vi "SLM_Azimuthal Generation.vi"(1 "p":i16 min=0 step=1, 2 "l":i16, 3 "beam parameters":T1={"amplitude matrix"=[], "number of columns in amplitude matrix"=128, "number of rows in amplitude matrix"=128, "represented width (in m)"=0.001, "represented height (in m)"=0.001, "wavelength (in m)"=6.33e-07} {"wavelength (in m)" format="%.2p"; "represented height (in m)" format="%.2p"; "represented width (in m)" format="%.2p"; "amplitude matrix" format="%.2f"}) -> (0 "Laguerre-Gaussian beam":T1 {"wavelength (in m)" format="%.2f"; "represented height (in m)" format="%.2f"; "represented width (in m)" format="%.2f"; "amplitude matrix" format="%.2f"})   [LabVIEW 2024]
panel:
  in  "y centre":dbl
  in  "x centre":dbl
  out "max value":dbl
  out "min value":dbl
  in  "beam waist w0 (in m; default 1E-4 = 0.1mm)":dbl=0.0001 format="%.2p"
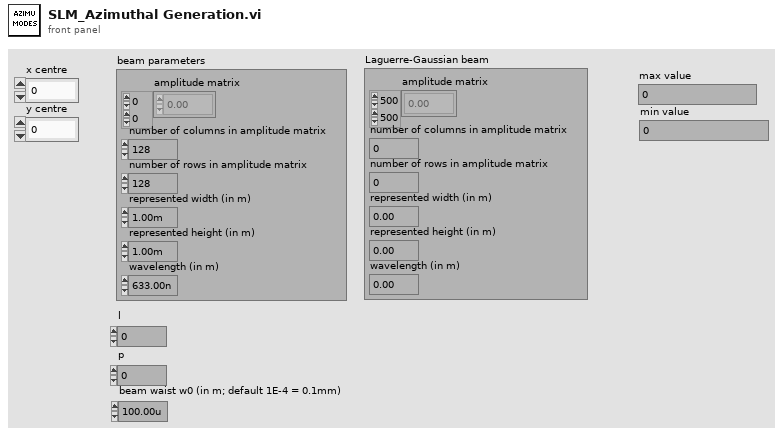
[diagram p1: front panel]
types:
  T1 = cluster{"amplitude matrix":csg[][], "number of columns in amplitude matrix":i32, "number of rows in amplitude matrix":i32, "represented width (in m)":dbl, "represented height (in m)":dbl, "wavelength (in m)":dbl}
  T2 = cluster{"x values":dbl[], "laguerre polynomial values":dbl[]}
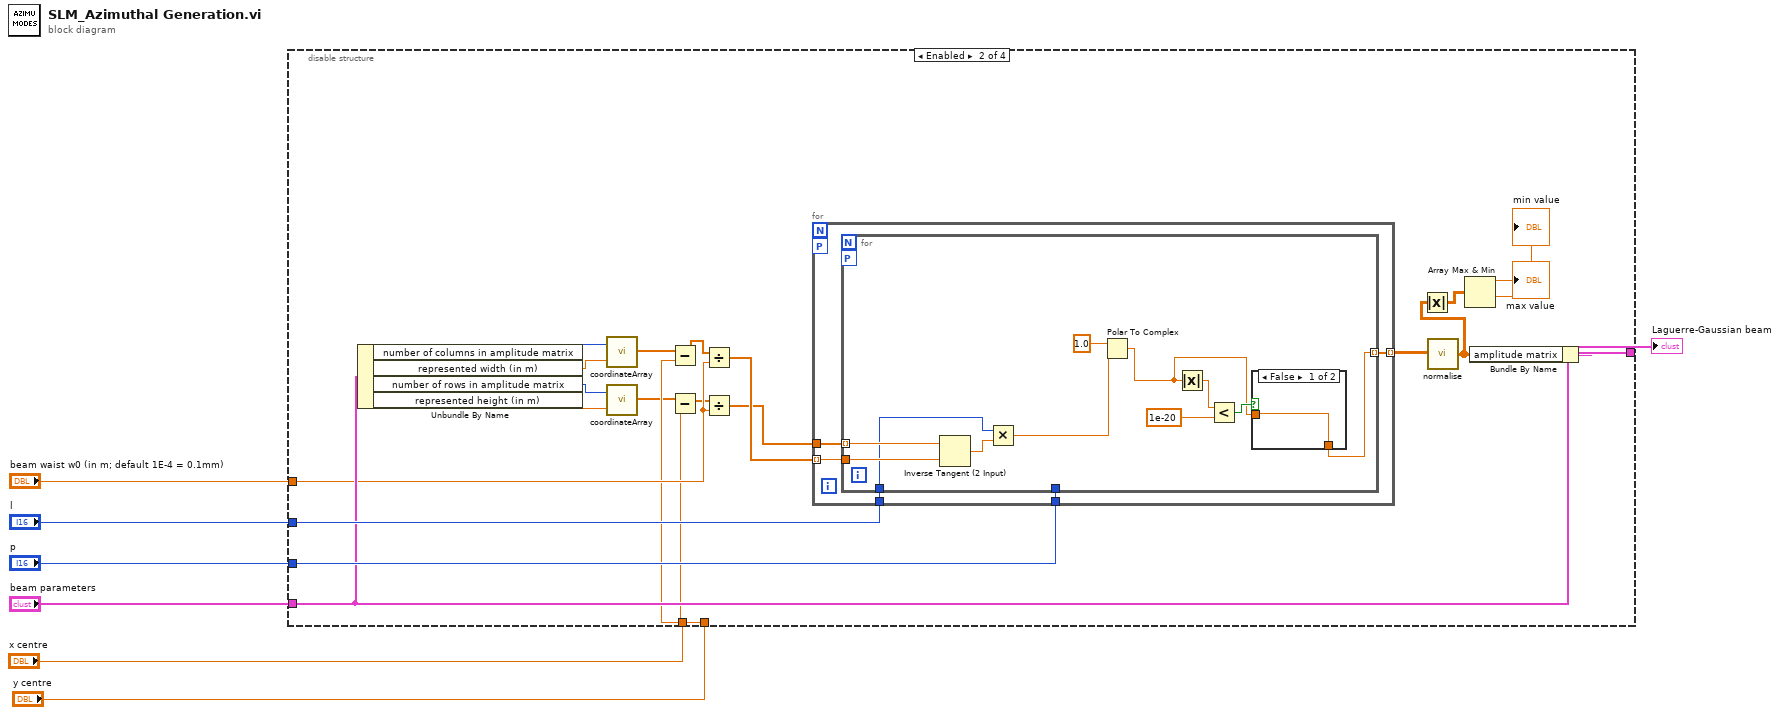
[diagram p0: block diagram]
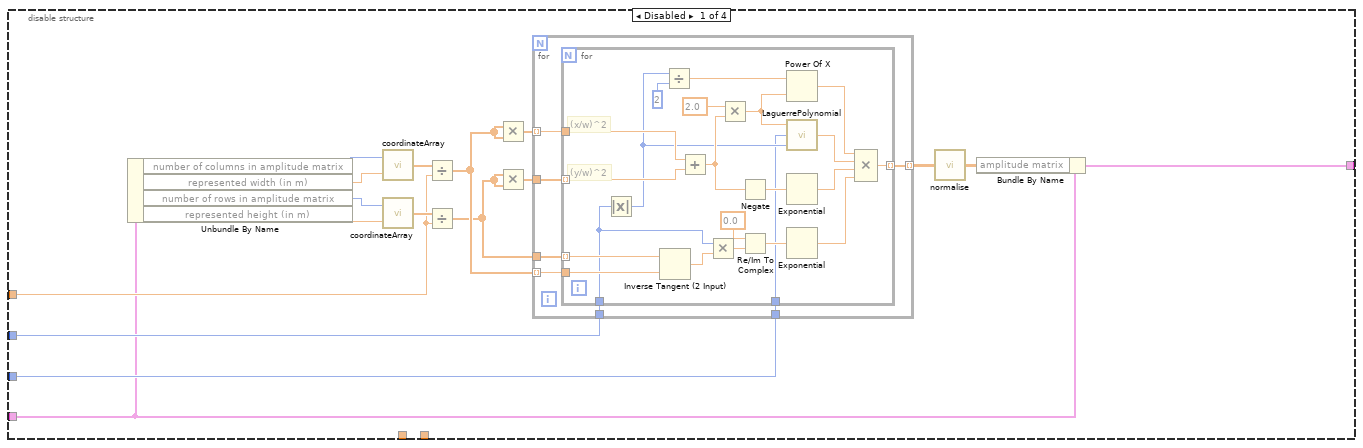
[diagram p2: hidden frame]
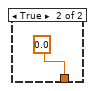
[diagram p3: hidden frame]
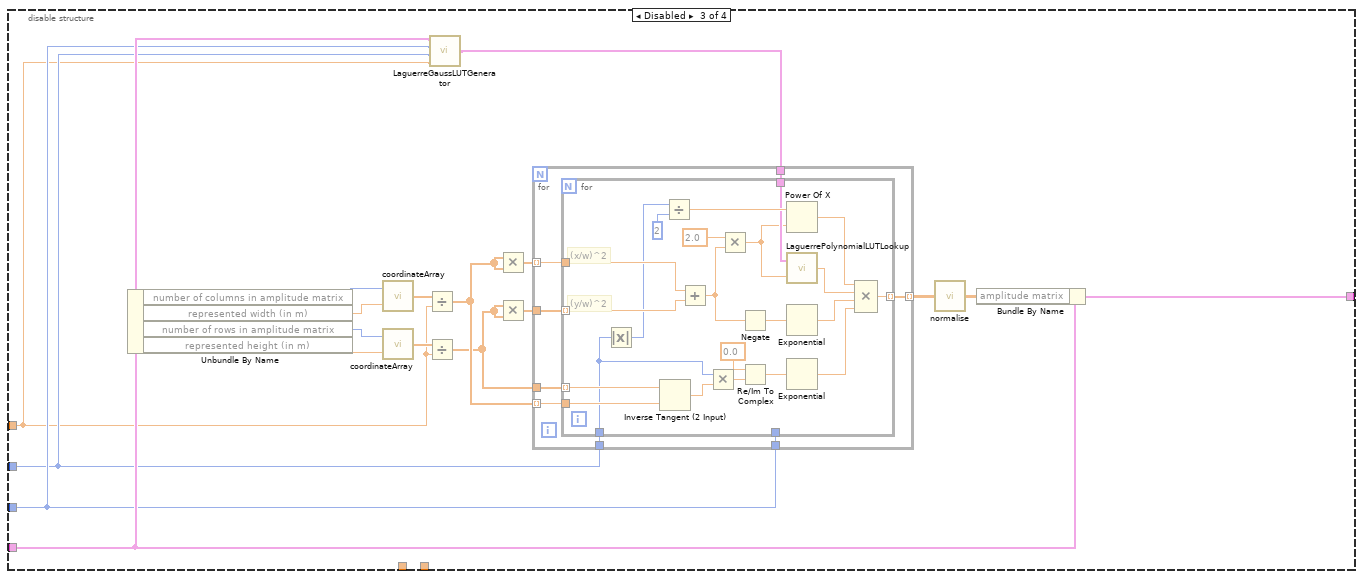
[diagram p4: hidden frame]
diagram:
  n1 = disable-structure shown="Enabled" {
    disable-tunnel: [w24 w75 w111 _] -> w7
    disable-tunnel: "p" -> [w11 w70 w96 _]
    disable-tunnel: "l" -> [w10 w69 w95 _]
    disable-tunnel: "beam waist w0 (in m; default 1E-4 = 0.1mm)" -> [w9 w67 w94 _]
    disable-tunnel: "beam parameters" -> [w8 w68 w97 _]
    disable-tunnel: "x centre" -> [_ w65 _ _]
    disable-tunnel: "y centre" -> [_ w66 _ _]
    frame Disabled {
      n2 = Unbundle By Name(w8) -> ("number of columns in amplitude matrix"=w23:i32, "represented width (in m)"=w13:dbl, "number of rows in amplitude matrix"=w22:i32, "represented height (in m)"=w12:dbl)
      n3 = call "coordinateArray.vi"("width of represented x (or y) range (in m; default 1E-3=1mm)"=w13, "array size (default 64)"=w23) -> ("x array"=w21:sgl[])
      n4 = call "coordinateArray.vi"("width of represented x (or y) range (in m; default 1E-3=1mm)"=w12, "array size (default 64)"=w22) -> ("x array"=w20:sgl[])
      n5 = Divide(x=w21, y=w9) -> (x/y=w17:dbl[])
      n6 = Divide(x=w20, y=w9) -> (x/y=w16:dbl[])
      n7 = Multiply(x=w17, y=w17) -> (x*y=w19:dbl[])
      n8 = Multiply(x=w16, y=w16) -> (x*y=w18:dbl[])
      n9 = for {
        tunnel: [w31] -> w15 mode=indexing
        tunnel: w19 -> [w30] mode=indexing
        tunnel: w18 -> [w29]
        tunnel: w17 -> [w28] mode=indexing
        tunnel: w16 -> [w27]
        tunnel: w10 -> [w26]
        tunnel: w11 -> [w25]
        n10 = for {
          tunnel: [w52] -> w31 mode=indexing
          tunnel: w30 -> [w51]
          tunnel: w29 -> [w50] mode=indexing
          tunnel: w28 -> [w40]
          tunnel: w27 -> [w39] mode=indexing
          tunnel: w26 -> [w36]
          tunnel: w25 -> [w32]
          # "(y/w)^2"
          # "(x/w)^2"
          n11 = Absolute Value(x=w36) -> (abs(x)=w33:i16)
          n12 = Inverse Tangent (2 Input)(1:w40, 2:w39) -> (0:w43:dbl)
          n13 = Divide(x=w33, y=i16 2) -> (x/y=w37:dbl)
          n14 = Add(x=w51, y=w50) -> (x+y=w47:dbl)
          n15 = Multiply(x=w36, y=w43) -> (x*y=w44:dbl)
          n16 = Multiply(x=2.0, y=w47) -> (x*y=w34:dbl)
          n17 = Negate(x=w47) -> (-x=w53:dbl)
          n18 = Re/Im To Complex(1:w44, 2:0.0 ("x")) -> (0:w45:cdb)
          n19 = Power Of X(1:w34, 2:w37) -> (0:w48:dbl)
          n20 = call "LaguerrePolynomial.vi"("a"=w33, "n"=w32, "x"=w34) -> ("associated Laguerre polynomial (n,a,x)"=w35:dbl)
          n21 = Exponential(1:w53) -> (0:w46:dbl)
          n22 = Exponential(1:w45) -> (0:w41:cdb)
          n23 = Compound Arithmetic op=MULTIPLY(w48, w35, w46, w41) -> (w52:cdb)
        }
      }
      n24 = call "normalise.vi"("amplitude matrix"=w15) -> ("normalised amplitude matrix"=w14:cdb[][])
      n25 = Bundle By Name(cluster=w8, "amplitude matrix"=w14) -> (w24:T1)
    }
    frame Enabled {
      n26 = Unbundle By Name(w68) -> ("number of columns in amplitude matrix"=w74:i32, "represented width (in m)"=w72:dbl, "number of rows in amplitude matrix"=w73:i32, "represented height (in m)"=w71:dbl)
      n27 = call "coordinateArray.vi"("width of represented x (or y) range (in m; default 1E-3=1mm)"=w72, "array size (default 64)"=w74) -> ("x array"=w64:sgl[])
      n28 = call "coordinateArray.vi"("width of represented x (or y) range (in m; default 1E-3=1mm)"=w71, "array size (default 64)"=w73) -> ("x array"=w61:sgl[])
      n29 = Subtract(x=w64, y=w65) -> (x-y=w60:dbl[])
      n30 = Subtract(x=w61, y=w66) -> (x-y=w59:dbl[])
      n31 = Divide(x=w60, y=w67) -> (x/y=w63:dbl[])
      n32 = Divide(x=w59, y=w67) -> (x/y=w62:dbl[])
      n33 = for {
        tunnel: [w80] -> w54 mode=indexing
        tunnel: w63 -> [w79] mode=indexing
        tunnel: w62 -> [w78]
        tunnel: w69 -> [w77]
        tunnel: w70 -> [w76]
        workers-P: _ -> [_]
        n34 = for {
          tunnel: [w83] -> w80 mode=indexing
          tunnel: w79 -> [w90]
          tunnel: w78 -> [w89] mode=indexing
          tunnel: w77 -> [w88]
          tunnel: w76 -> [_]
          workers-P: _ -> [_]
          n35 = Inverse Tangent (2 Input)(1:w90, 2:w89) -> (0:w91:dbl)
          n36 = Multiply(x=w88, y=w91) -> (x*y=w87:dbl)
          n37 = Polar To Complex(1:w87, 2:1.0 ("r")) -> (0:w81:cdb)
          n38 = Absolute Value(x=w81) -> (abs(x)=w86:dbl)
          n39 = Less?(x=w86, y=1e-20) -> (x < y?=w84:bool)
          n40 = case shown="False" w84 {
            tunnel: w81 -> [w92 _]
            tunnel: [w92 0.0 ("y")] -> w83
            frame False {
            }
            frame True {
            }
          }
        }
      }
      n41 = call "normalise.vi"("amplitude matrix"=w54) -> ("normalised amplitude matrix"=w55:cdb[][])
      n42 = Absolute Value(x=w55) -> (abs(x)=w58:dbl[][])
      n43 = Array Max & Min(array=w58) -> (max value=→"max value":dbl, min value=→"min value":dbl)  [unwired: 2 out]
      n44 = Bundle By Name(cluster=w68, "amplitude matrix"=w55) -> (w75:T1)
    }
    frame Disabled {
      n45 = Unbundle By Name(w97) -> ("number of columns in amplitude matrix"=w110:i32, "represented width (in m)"=w100:dbl, "number of rows in amplitude matrix"=w109:i32, "represented height (in m)"=w99:dbl)
      n46 = call "coordinateArray.vi"("width of represented x (or y) range (in m; default 1E-3=1mm)"=w100, "array size (default 64)"=w110) -> ("x array"=w108:sgl[])
      n47 = call "coordinateArray.vi"("width of represented x (or y) range (in m; default 1E-3=1mm)"=w99, "array size (default 64)"=w109) -> ("x array"=w107:sgl[])
      n48 = Divide(x=w108, y=w94) -> (x/y=w104:dbl[])
      n49 = Divide(x=w107, y=w94) -> (x/y=w103:dbl[])
      n50 = call "LaguerreGaussLUTGenerator.vi"("beam waist w0 (in m; default 1E-4 = 0.1mm)"=w94, "l"=w95, "p"=w96, "beam parameters"=w97) -> ("Look-up Table"=w98:T2)
      n51 = Multiply(x=w104, y=w104) -> (x*y=w106:dbl[])
      n52 = Multiply(x=w103, y=w103) -> (x*y=w105:dbl[])
      n53 = for {
        tunnel: [w119] -> w102 mode=indexing
        tunnel: w106 -> [w118] mode=indexing
        tunnel: w105 -> [w117]
        tunnel: w104 -> [w116] mode=indexing
        tunnel: w103 -> [w115]
        tunnel: w95 -> [w114]
        tunnel: w96 -> [w113]
        tunnel: w98 -> [w112]
        n54 = for {
          tunnel: [w140] -> w119 mode=indexing
          tunnel: w118 -> [w139]
          tunnel: w117 -> [w138] mode=indexing
          tunnel: w116 -> [w128]
          tunnel: w115 -> [w127] mode=indexing
          tunnel: w114 -> [w124]
          tunnel: w113 -> [_]
          tunnel: w112 -> [w122]
          # "(y/w)^2"
          # "(x/w)^2"
          n55 = Absolute Value(x=w124) -> (abs(x)=w123:i16)
          n56 = Inverse Tangent (2 Input)(1:w128, 2:w127) -> (0:w131:dbl)
          n57 = Divide(x=w123, y=i16 2) -> (x/y=w125:dbl)
          n58 = Add(x=w139, y=w138) -> (x+y=w135:dbl)
          n59 = Multiply(x=w124, y=w131) -> (x*y=w132:dbl)
          n60 = Multiply(x=2.0, y=w135) -> (x*y=w121:dbl)
          n61 = Negate(x=w135) -> (-x=w141:dbl)
          n62 = Re/Im To Complex(1:w132, 2:0.0 ("x")) -> (0:w133:cdb)
          n63 = Power Of X(1:w121, 2:w125) -> (0:w136:dbl)
          n64 = call "LaguerrePolynomialLUTLookup.vi"("x"=w121, "Look-up Table"=w122) -> ("Function value"=w120:dbl)
          n65 = Exponential(1:w141) -> (0:w134:dbl)
          n66 = Exponential(1:w133) -> (0:w129:cdb)
          n67 = Compound Arithmetic op=MULTIPLY(w136, w120, w134, w129) -> (w140:cdb)
        }
      }
      n68 = call "normalise.vi"("amplitude matrix"=w102) -> ("normalised amplitude matrix"=w101:cdb[][])
      n69 = Bundle By Name(cluster=w97, "amplitude matrix"=w101) -> (w111:T1)
    }
    frame Disabled {
    }
  }
  "Laguerre-Gaussian beam" <- w7
